vi "dT.vi"(8 "error in":errorcluster, 11 "Old Time":dbl) -> (0 "error out":errorcluster, 2 "dT (ms)":dbl, 3 "New Time":dbl format="%_19f")   [LabVIEW 2024]
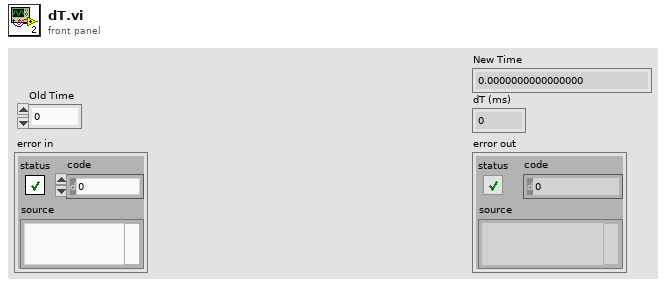
[diagram p1: front panel]
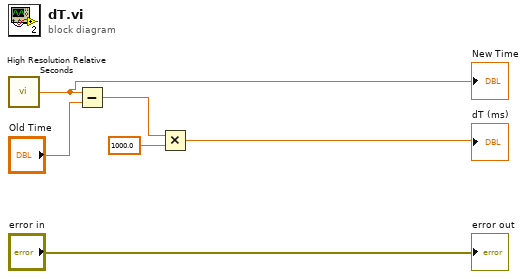
[diagram p0: block diagram]
diagram:
  n1 = call <vilib>:"High Resolution Relative Seconds.vi"() -> ("relative seconds"=w5:dbl)
  "New Time" <- w5
  n2 = Subtract(x=w5, y="Old Time") -> (x-y=w4:dbl)
  n3 = Multiply(x=w4, y=1000.0) -> (x*y=→"dT (ms)":dbl)
  "error out" <- "error in"
